vi "GetType.vi"(8 "Error In":errorcluster, 11 "reference in":refnum<class "VdDigitalControl.lvclass">) -> (0 "Error Out":errorcluster, 2 "InstrumentType":T1, 3 "reference in":refnum<class "VdDigitalControl.lvclass">)   [LabVIEW 2020, in "VdDigitalControl.lvclass"]
uses:
  VdDigitalControl.lvclass
  VdDigitalControl.lvclass/VdDigitalControl.ctl
  VdInstrument_class/InstrumentType.ctl
  VdInstrument_class/VdInstrument.lvclass
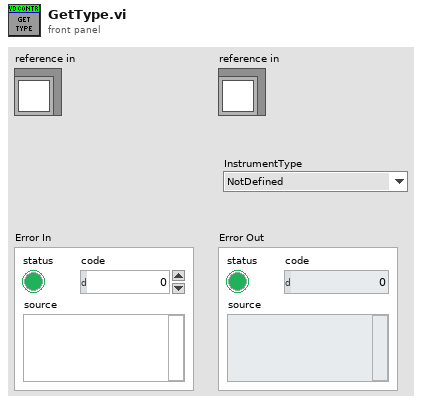
[diagram p1: front panel]
types:
  T1 = typedef "VdInstrument.lvclass/InstrumentType.ctl" = enum16{"NotDefined", "AirflowController", "AnalogInput", "AnalogOutput", "AutoCollimator", "BeamProfiler", "DMM", "DigitalControl", "DigitalInput", "DisplacementSensor", "Encoder", "ForceSensor", "FrequencyCounter", "FunctionGenerator", "GelDispensingRobot", "GlueDispenser", "Hexapod", "IRCamera", "ImageGenerator", "LabelPrinter", "LightController", "LightIndicator", "Load", "Multimeter", "OpticalAttenuatorPowerMeter", "OpticalChannelMonitor", "OpticalLaser", "OpticalPolarizationController", "OpticalPowerAttenuator", "OpticalPowerMeter", "OpticalSpectrumAnalyzer", "PDLMeter", "PolarisationScrambler", "PolarizationAnalyzer", "PositionSensitiveDetector", "PowerSupply", "PressureController", "Robot", "SLRCamera", "ScrewdriverController", "SignalAnalyzer", "SignalGenerator", "SixAxisStage", "SolderingStation", "SpectrumAnalyzer", "StepperMotor", "Stirrer", "SweptWavelengthSystem", "Switch", "TemperatureChamber", "TemperatureController", "TemperatureSensor", "TunableLaser", "UVCuring", "UsbHub", "VisionCamera", "WavelengthMeter", "WeldingLaser"}
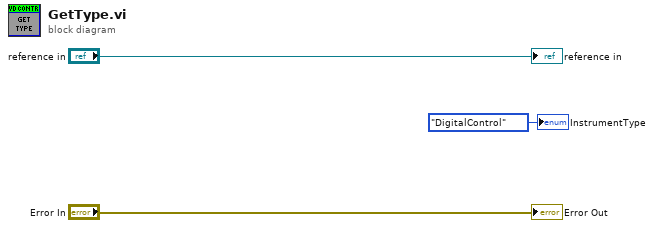
[diagram p0: block diagram]
diagram:
  "Error Out" <- "Error In"
  "reference in" <- "reference in"
  "InstrumentType" <- InstrumentType."DigitalControl" ("InstrumentType")
